vi "stopped.vi"(8 "error in (no error)":errorcluster, 10 "stopped":bool, 11 "WinX32Camera in":refnum<class "WinX32Camera.lvclass">) -> (0 "error out":errorcluster, 3 "WinX32Camera out":refnum<class "WinX32Camera.lvclass">)   [LabVIEW 2011, in "WinX32Camera.lvclass"]
uses:
  WinX32Camera.lvclass
  WinX32Camera.lvclass/WinX32Camera.ctl
panel:
  # "gets called on the control computer, by the\nimaging computer."
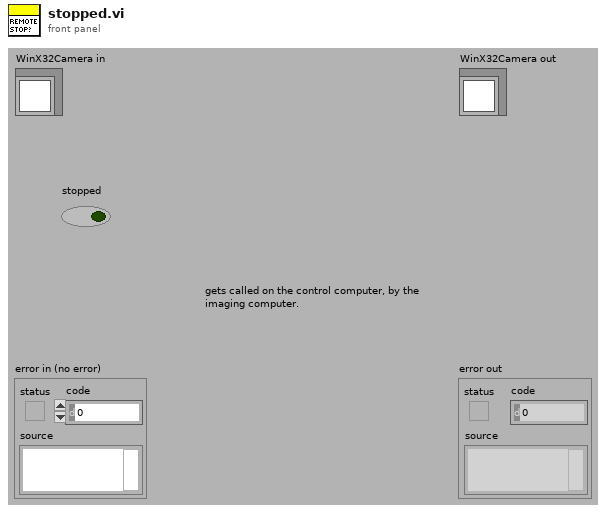
[diagram p1: front panel]
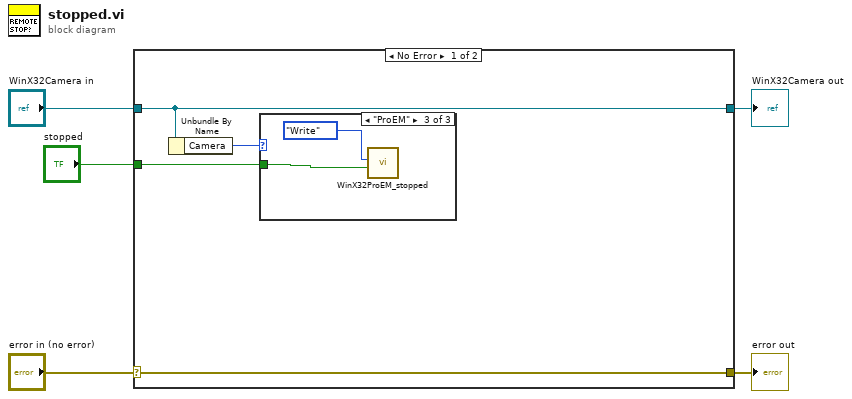
[diagram p0: block diagram]
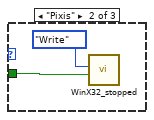
[diagram p3: hidden frame]
diagram:
  n1 = case shown="No Error" "error in (no error)" {
    selector: "error in (no error)" -> [w9 w15]
    tunnel: [w9 w15] -> w4
    tunnel: [w7 w14] -> w2
    tunnel: "WinX32Camera in" -> [w7 w14]
    tunnel: "stopped" -> [w8 _]
    frame No Error {
      n2 = Unbundle By Name(w7) -> ("Camera"=w6:enum16{"Simulation", "Pixis", "ProEM"})
      n3 = case shown="\"ProEM\"" w6 {
        tunnel: w8 -> [_ w11 w12]
        frame "Simulation", Default {
        }
        frame "Pixis" {
          n4 = call "WinX32_stopped.vi"("stop"=w11, "Action"=enum16{"Write", "Read"}."Write") -> ()  [unwired: 9 in, 1 out]
        }
        frame "ProEM" {
          n5 = call "WinX32ProEM_stopped.vi"("stop"=w12, "Action"=enum16{"Write", "Read"}."Write") -> ()  [unwired: 9 in, 1 out]
        }
      }
    }
    frame Error {
    }
  }
  "error out" <- w4
  "WinX32Camera out" <- w2
